vi "poly_data_queue_ArrayFXP.vi"(5 "skip? (F)":bool, 6 "initial queue element (vector of NaNs)":fxp<+/-,64,32>[](array[numeric]), 7 "initialize":bool, 8 "error in":errorcluster caption="Error in (no error)", 9 "queue length (100)":i32=100, 10 "input data element":fxp<+/-,64,32>[](array[numeric])) -> (0 "error out":errorcluster, 1 "eliminated element":fxp<+/-,64,32>[](array[numeric]), 2 "queue":fxp<+/-,64,32>[][](array[numeric]), 4 "current length":i32)   [LabVIEW 2015]
uses:
  poly_average_tools_eco_plus.vi
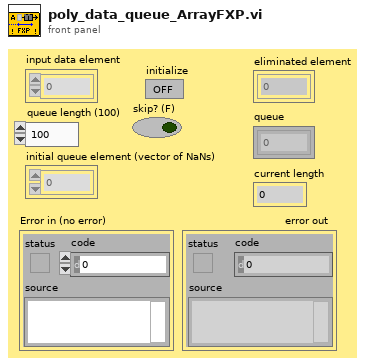
[diagram p1: front panel]
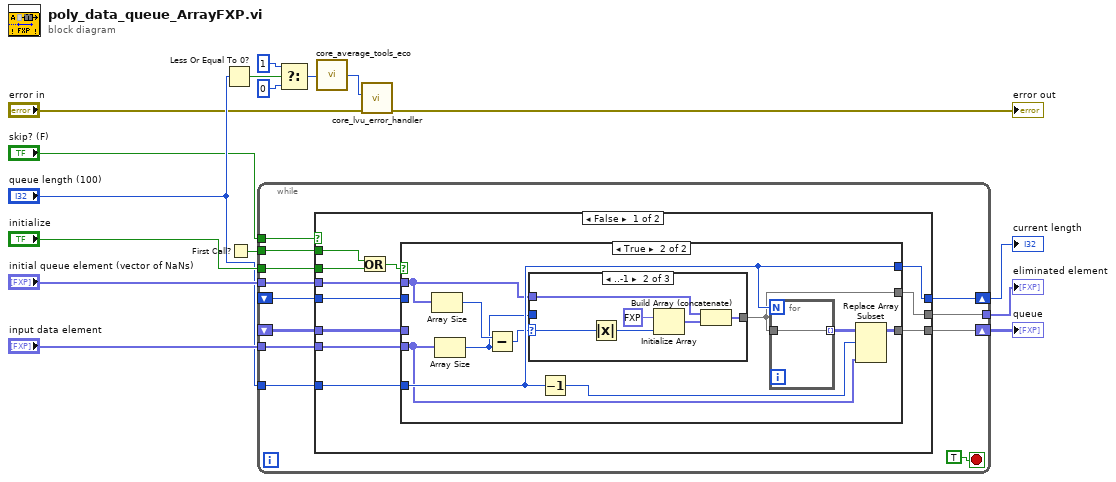
[diagram p0: block diagram]
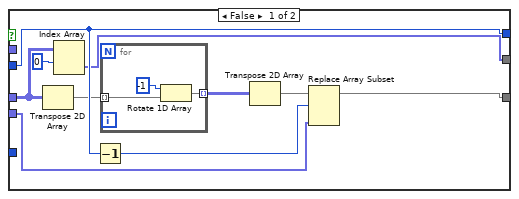
[diagram p2: hidden frame]
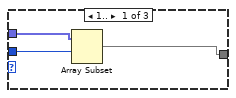
[diagram p3: hidden frame]
diagram:
  n1 = Less Or Equal To 0?(x="queue length (100)") -> (x <= 0?=w9:bool)
  n2 = First Call?() -> (First Call?: T/F=w10:bool)
  n3 = while {
    tunnel: w10 -> [w23]
    shift-left: _ -> [w26]
    shift-right: [w27] -> w16
    shift-left: _ -> [w25]
    shift-right: [w28] -> w4
    tunnel: "initialize" -> [w22]
    tunnel: "input data element" -> [w21]
    tunnel: "initial queue element (vector of NaNs)" -> [w20]
    tunnel: "queue length (100)" -> [w19]
    tunnel: [w18] -> w12
    tunnel: "skip? (F)" -> [w17]
    stop <- TRUE stop-if-true
    n4 = case shown="False" w17 {
      tunnel: [w39 w76] -> w28
      tunnel: [w38 w74] -> w27
      tunnel: w26 -> [w37 w74]
      tunnel: w25 -> [w36 w76]
      tunnel: w23 -> [w35 _]
      tunnel: w22 -> [w33 _]
      tunnel: w21 -> [w32 w75]
      tunnel: w20 -> [w31 _]
      tunnel: w19 -> [w30 _]
      tunnel: [w29 w75] -> w18
      frame False {
        n5 = Or(x=w35, y=w33) -> (x .or. y?=w34:bool)
        n6 = case shown="True" w34 {
          tunnel: [w47 w61] -> w39
          tunnel: [w48 w60] -> w38
          tunnel: w37 -> [w48 _]
          tunnel: w36 -> [w41 _]
          tunnel: w32 -> [w49 w58]
          tunnel: w31 -> [_ w57]
          tunnel: w30 -> [_ w60]
          tunnel: [w44 w56] -> w29
          frame False {
            n7 = Transpose 2D Array(2D array=w41) -> (transposed array=w43:fxp<+/-,64,32>[][])
            n8 = Index Array(array=w41, index (row)=0 ("Index")) -> (element=w44:fxp<+/-,64,32>[])  [unwired: 1 in]
            n9 = Decrement(x=w48) -> (x-1=w46:i32)
            n10 = for {
              tunnel: w43 -> [w52] mode=indexing
              tunnel: [w51] -> w42 mode=indexing
              n11 = Rotate 1D Array(1:w52, 2:i16 -1 ("n")) -> (0:w51:fxp<+/-,64,32>[])
            }
            n12 = Transpose 2D Array(2D array=w42) -> (transposed array=w40:fxp<+/-,64,32>[][])
            n13 = Replace Array Subset(array=w40, new element=w49, index (row)=w46) -> (w47:fxp<+/-,64,32>[][])  [unwired: 1 in]
          }
          frame True {
            n14 = Array Size(array=w57) -> (size(s)=w55:i32)
            n15 = Array Size(array=w58) -> (size(s)=w53:i32)
            n16 = Subtract(x=w55, y=w53) -> (x-y=w54:i32)
            n17 = case shown="..-1" w54 {
              selector: w54 -> [_ w71 _]
              tunnel: [w63 w66 w72] -> w56
              tunnel: w57 -> [w65 w68 w72]
              tunnel: w53 -> [w64 _ _]
              frame 1.. {
                n18 = Array Subset(array=w65, index=w64) -> (w63:fxp<+/-,64,32>[])  [unwired: 1 in]
              }
              frame ..-1 {
                n19 = Absolute Value(x=w71) -> (abs(x)=w70:i32)
                n20 = Initialize Array(fxp<+,1,1> 0.0 ("element"), w70) -> (w67:fxp<+,1,1>[])
                n21 = Build Array (concatenate)(w68, w67) -> (w66:fxp<+/-,64,32>[])
              }
              frame 0 {
              }
            }
            n22 = Decrement(x=w60) -> (x-1=w62:i32)
            n23 = for {
              N: w60 -> [_]
              tunnel: w56 -> [w73]
              tunnel: [w73] -> w59 mode=indexing
            }
            n24 = Replace Array Subset(array=w59, new element=w58, index (row)=w62) -> (w61:fxp<+/-,64,32>[][])  [unwired: 1 in]
          }
        }
      }
      frame True {
      }
    }
  }
  "queue" <- w4
  "current length" <- w16
  "eliminated element" <- w12
  n25 = Select(t=1, s=w9, f=0) -> (s? t:f=w2:i32)
  n26 = call-poly "core_average_tools_eco.vi"("code (w/out eco)"=w2) -> ("code (+ eco)"=w1:i32)  [unwired: 4 in]
  n27 = call "core_lvu_error_handler.vi"("error in (no error)"="error in", "code (0 = no error)"=w1) -> ("error out"=→"error out":errorcluster)  [unwired: 8 in, 1 out]
